vi "Creating an Array.vi"() -> ()   [LabVIEW 2015]
uses:
  Title - Type Def.ctl
  Employee Record - Type Def.ctl
panel:
  in  "Employee Record":T1[](array[typedef]) {"Start Date" format="%<%x %.3X>T"}
  in  "Numeric Array":dbl[](array[numeric])
  in  "Numeric":dbl
  in  "Array":void[](array[numeric])
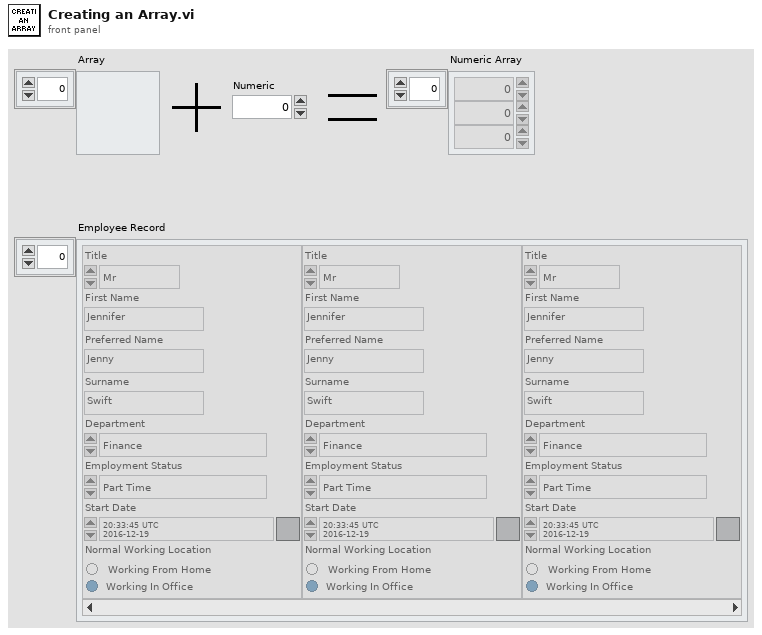
[diagram p1: front panel]
types:
  T1 = typedef "Employee Record - Type Def.ctl" = cluster{"Title":T2, "First Name":string, "Preferred Name":string, "Surname":string, "Department":enum16{"Research and Development", "Technical Support", "Sales", "Management", "Finance", "Other"}, "Employment Status":enum16{"Full Time", "Part Time", "No Longer Employed", "Probation", "Other"}, "Start Date":timestamp, "Normal Working Location":enum32{"Working From Home", "Working in Office"}}
  T2 = typedef "Title - Type Def.ctl" = enum16{"Mr", "Mrs", "Ms", "Mx", "Miss", "Sir", "Dame", "Other"}
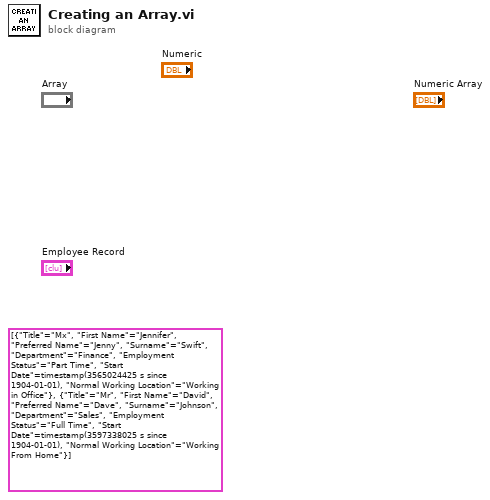
[diagram p0: block diagram]
diagram:
  (unwired) T1[] [{"Title"=enum."Mx", "First Name"="Jennifer", "Preferred Name"="Jenny", "Surname"="Swift", "Department"=enum."Finance", "Employment Status"=enum."Part Time", "Start Date"=timestamp(3565024425.501588 s since 1904-01-01), "Normal Working Location"=enum."Working in Office"}, {"Title"=enum."Mr", "First Name"="David", "Preferred Name"="Dave", "Surname"="Johnson", "Department"=enum."Sales", "Employment Status"=enum."Full Time", "Start Date"=timestamp(3597338025.501588 s since 1904-01-01), "Normal Working Location"=enum."Working From Home"}] ("Employee Record")
